vi "Dashboard.vi"() -> ()   [LabVIEW 2013]
uses:
  2014 Robot Project/Robot Global Data.vi
  <vilib>/sound2/lvsound2.llb/Sound File Read Open.vi
  <vilib>/sound2/lvsound2.llb/Sound File Read (DBL).vi
panel:
  out "Feeder":bool
  out "InvertDrive":bool
  out "ThumpFire":bool
  out "ThumpHigh":bool
  out "ThumpLow":bool
  out "DownLimit":bool
  out "DownLimit 2":bool
  out "Center":bool
  out "UpLimit 2":bool
  out "UpLimit":bool
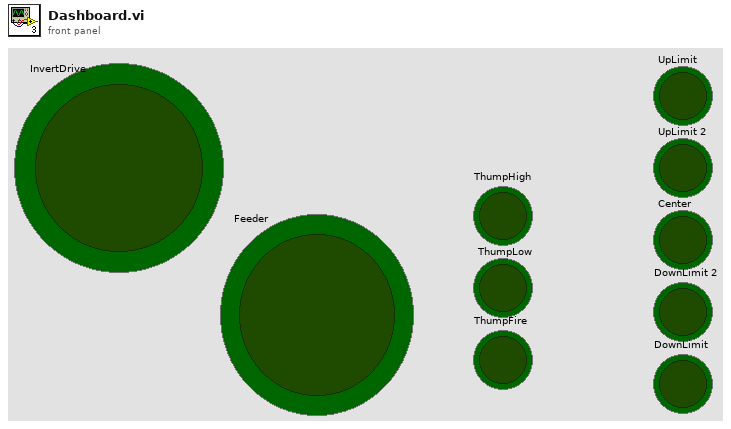
[diagram p1: front panel]
types:
  T1 = cluster{"UpLimit":bool, "Up2":bool, "Center":bool, "Down2":bool, "DownLimit":bool, "ThumpState":dbl, "ShifterState":bool, "FeederState":bool}
  T2 = cluster{"Competition mode":bool, "Robot Link":bool, "Autonomous":bool, "Enabled":bool, "E-Stop":bool, "Simulated":bool, "TestMode":bool, "Docked Window":bool}
  T3 = typedef "Sound File Refnum.ctl" = refnum<file>
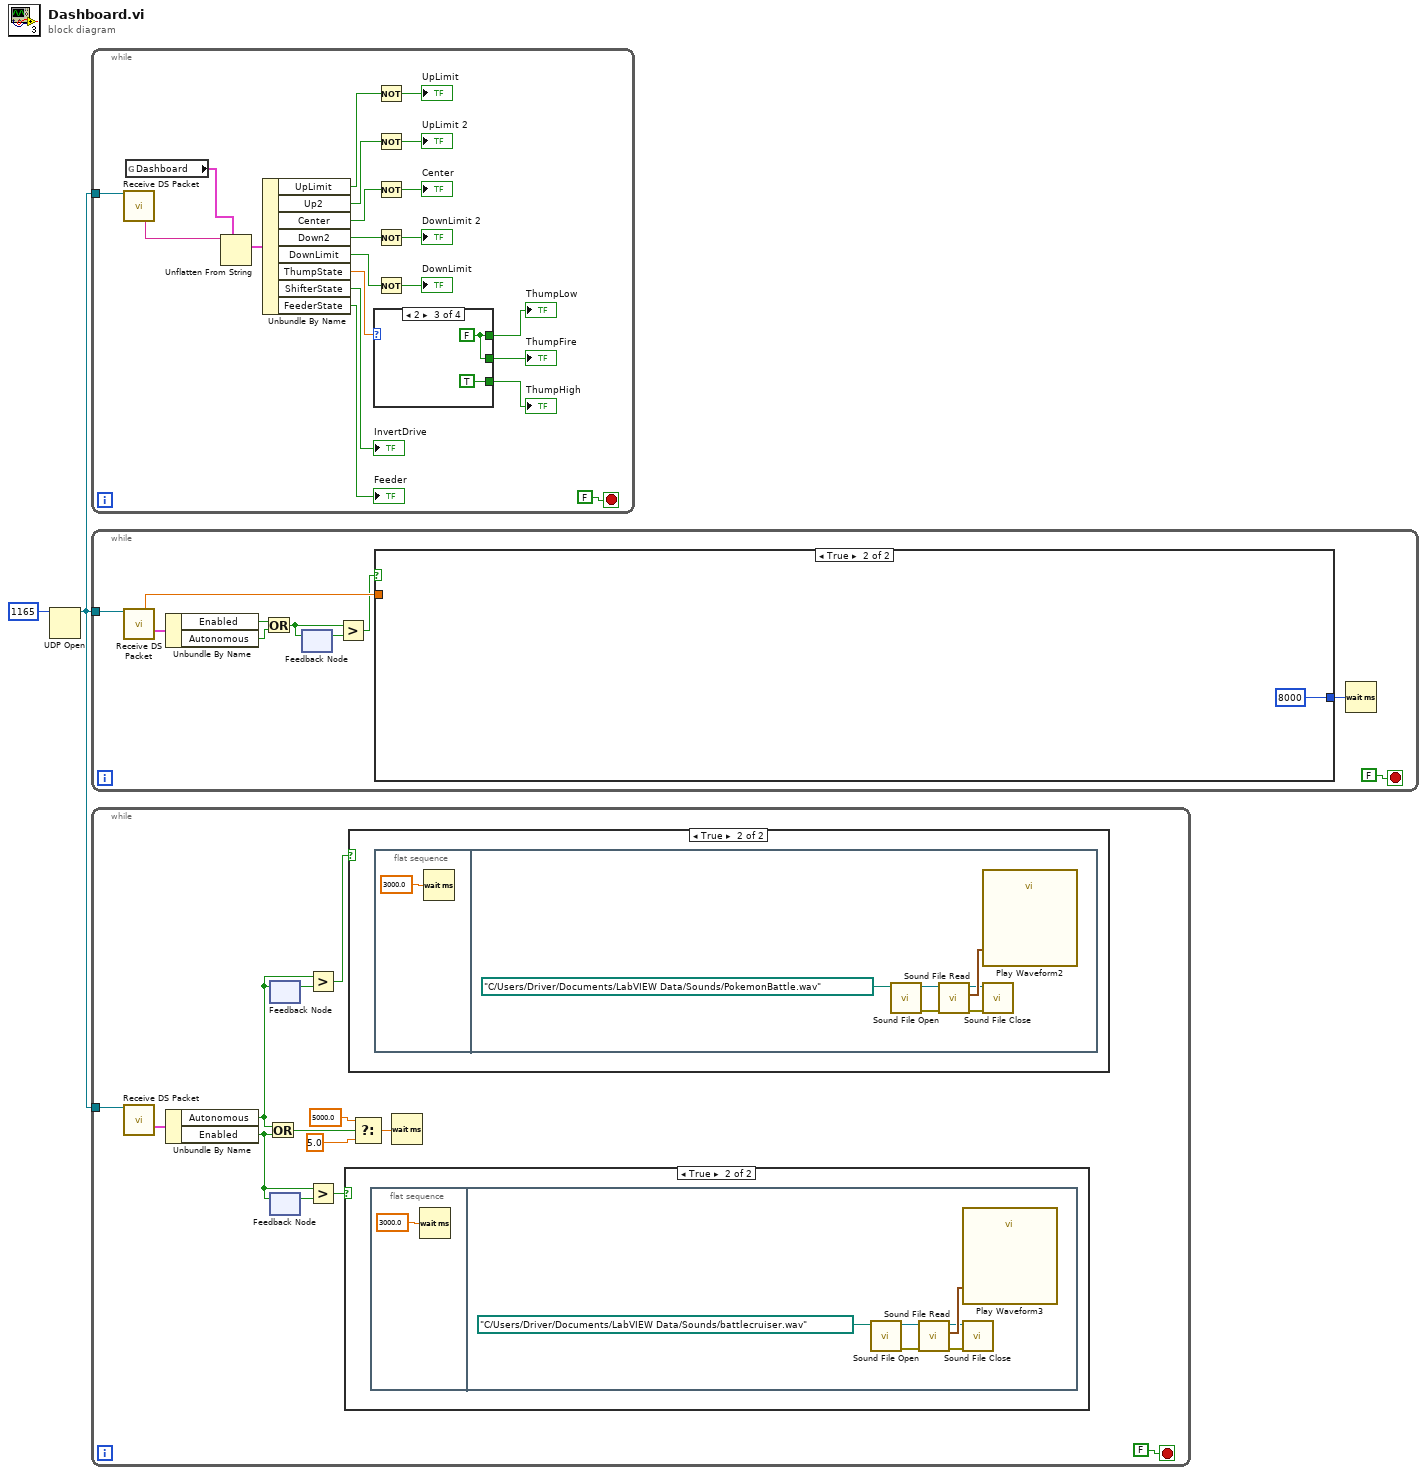
[diagram p0: block diagram]
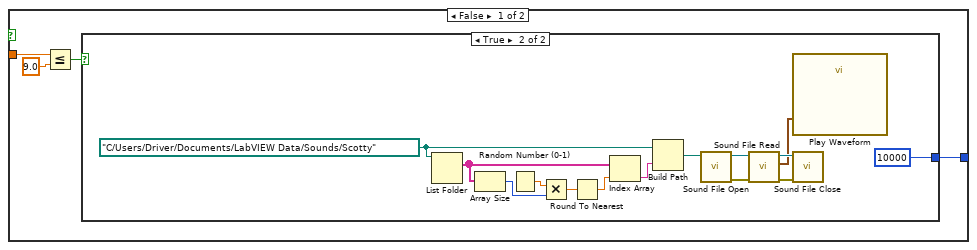
[diagram p4: hidden frame]
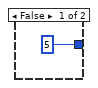
[diagram p5: hidden frame]
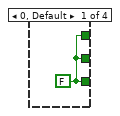
[diagram p6: hidden frame]
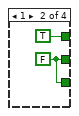
[diagram p7: hidden frame]
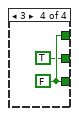
[diagram p8: hidden frame]
diagram:
  n1 = UDP Open(11:u16 1165 ("port")) -> (port=w1:refnum<k16>)  [unwired: 4 in, 2 out]
  n2 = while {
    tunnel: w1 -> [w23]
    stop <- FALSE stop-if-true
    n3 = call "Receive DS Packet.vi"("Recv Socket"=w23) -> ("High Priority User Data"=w22:string)  [unwired: 5 in, 9 out]
    n4 = global read "Robot Global Data.vi" "Dashboard"() -> (w20:T1)
    n5 = Unflatten From String(type=w20, binary string=w22) -> (value=w19:T1)  [unwired: 3 in, 2 out]
    n6 = Unbundle By Name(w19) -> ("UpLimit"=w7:bool, "Up2"=w6:bool, "Center"=w5:bool, "Down2"=w4:bool, "DownLimit"=w3:bool, "ThumpState"=w16:dbl, "ShifterState"=→"InvertDrive":bool, "FeederState"=→"Feeder":bool)
    n7 = case shown="2" w16 {
      tunnel: [w24 w26 TRUE w30] -> w15
      tunnel: [w24 TRUE w28 w30] -> w14
      tunnel: [w24 w26 w28 TRUE] -> w13
      frame 0, Default {
        w24 = FALSE
      }
      frame 1 {
        w26 = FALSE
      }
      frame 2 {
        w28 = FALSE
      }
      frame 3 {
        w30 = FALSE
      }
    }
    "ThumpHigh" <- w15
    "ThumpFire" <- w13
    "ThumpLow" <- w14
    n8 = Not(x=w7) -> (.not. x?=→"UpLimit":bool)
    n9 = Not(x=w6) -> (.not. x?=→"UpLimit 2":bool)
    n10 = Not(x=w5) -> (.not. x?=→"Center":bool)
    n11 = Not(x=w4) -> (.not. x?=→"DownLimit 2":bool)
    n12 = Not(x=w3) -> (.not. x?=→"DownLimit":bool)
  }
  n13 = while {
    tunnel: w1 -> [w40]
    stop <- FALSE stop-if-true
    n14 = call "Receive DS Packet.vi"("Recv Socket"=w40) -> ("Battery"=w39:sgl, "Status"=w36:T2)  [unwired: 5 in, 8 out]
    n15 = Unbundle By Name(w36) -> ("Enabled"=w33:bool, "Autonomous"=w32:bool)
    n16 = Or(x=w33, y=w32) -> (x .or. y?=w31:bool)
    n17 = feedback-in #1(w31) -> ()
    n18 = feedback #1() -> (w35:bool)  [unwired: 1 in]
    n19 = Greater?(x=w31, y=w35) -> (0:w34:bool)
    n20 = case shown="True" w34 {
      tunnel: w39 -> [w42 _]
      tunnel: [w41 8000] -> w38
      frame False {
        n21 = Less Or Equal?(x=w42, y=sgl 9.0) -> (x <= y?=w43:bool)
        n22 = case shown="True" w43 {
          tunnel: [5 10000] -> w41
          frame False {
          }
          frame True {
            w54 = path "C:/Users/Driver/Documents/LabVIEW Data/Sounds/Scotty" ("path")
            n23 = List Folder(path=w54) -> (filenames=w55:string[])  [unwired: 3 in, 3 out]
            n24 = Array Size(array=w55) -> (size(s)=w58:i32)
            n25 = Random Number (0-1)() -> (number: 0 to 1=w59:dbl)
            n26 = Multiply(x=w59, y=w58) -> (x*y=w57:dbl)
            n27 = Round To Nearest(number=w57) -> (nearest integer value=w56:dbl)
            n28 = Index Array(array=w55, index=w56) -> (element=w53:string)
            n29 = Build Path(base path=w54, name or relative path=w53) -> (appended path=w52:path)
            n30 = call-poly <vilib>:"Sound File Open.vi"("path"=w52) -> ("error out"=w48:errorcluster, "sound file refnum"=w51:T3)  [unwired: 9 in]
            n31 = call-poly <vilib>:"Sound File Read.vi"("error in (no error)"=w48, "sound file refnum"=w51) -> ("error out"=w49:errorcluster, "data"=w47:waveform(dbl)[], "sound file refnum out"=w50:T3)  [unwired: 5 in, 2 out]
            n32 = call "Play Waveform"("Data"=w47) -> ()  [unwired: 18 in, 1 out]
            n33 = call <vilib>:"Sound File Close.vi"("error in (no error)"=w49, "sound file refnum"=w50) -> ()  [unwired: 9 in, 1 out]
          }
        }
      }
      frame True {
      }
    }
    n34 = Wait (ms)(milliseconds to wait=w38) -> ()  [unwired: 1 out]
  }
  n35 = while {
    tunnel: w1 -> [w61]
    stop <- FALSE stop-if-true
    n36 = call "Receive DS Packet.vi"("Recv Socket"=w61) -> ("Status"=w73:T2)  [unwired: 5 in, 9 out]
    n37 = Unbundle By Name(w73) -> ("Autonomous"=w67:bool, "Enabled"=w66:bool)
    n38 = Or(x=w67, y=w66) -> (x .or. y?=w65:bool)
    n39 = feedback #2() -> (w72:bool)  [unwired: 1 in]
    n40 = feedback-in #2(w67) -> ()
    n41 = feedback #3() -> (w69:bool)  [unwired: 1 in]
    n42 = feedback-in #3(w66) -> ()
    n43 = Greater?(x=w67, y=w72) -> (0:w70:bool)
    n44 = Greater?(x=w66, y=w69) -> (0:w68:bool)
    n45 = case shown="True" w68 {
      frame False {
      }
      frame True {
        n46 = flat-sequence {
          frame #0 {
            n47 = Wait (ms)(milliseconds to wait=3000.0 ("t")) -> ()  [unwired: 1 out]
          }
          frame #1 {
            n48 = call-poly <vilib>:"Sound File Open.vi"("path"=path "C:/Users/Driver/Documents/LabVIEW Data/Sounds/battlecruiser.wav") -> ("error out"=w78:errorcluster, "sound file refnum"=w75:T3)  [unwired: 9 in]
            n49 = call-poly <vilib>:"Sound File Read.vi"("error in (no error)"=w78, "sound file refnum"=w75) -> ("error out"=w77:errorcluster, "data"=w79:waveform(dbl)[], "sound file refnum out"=w76:T3)  [unwired: 5 in, 2 out]
            n50 = call "Play Waveform3"("Data"=w79) -> ()  [unwired: 18 in, 1 out]
            n51 = call <vilib>:"Sound File Close.vi"("error in (no error)"=w77, "sound file refnum"=w76) -> ()  [unwired: 9 in, 1 out]
          }
        }
      }
    }
    n52 = case shown="True" w70 {
      frame False {
      }
      frame True {
        n53 = flat-sequence {
          frame #0 {
            n54 = Wait (ms)(milliseconds to wait=3000.0 ("t")) -> ()  [unwired: 1 out]
          }
          frame #1 {
            n55 = call-poly <vilib>:"Sound File Open.vi"("path"=path "C:/Users/Driver/Documents/LabVIEW Data/Sounds/PokemonBattle.wav") -> ("error out"=w85:errorcluster, "sound file refnum"=w82:T3)  [unwired: 9 in]
            n56 = call-poly <vilib>:"Sound File Read.vi"("error in (no error)"=w85, "sound file refnum"=w82) -> ("error out"=w84:errorcluster, "data"=w86:waveform(dbl)[], "sound file refnum out"=w83:T3)  [unwired: 5 in, 2 out]
            n57 = call "Play Waveform2"("Data"=w86) -> ()  [unwired: 18 in, 1 out]
            n58 = call <vilib>:"Sound File Close.vi"("error in (no error)"=w84, "sound file refnum"=w83) -> ()  [unwired: 9 in, 1 out]
          }
        }
      }
    }
    n59 = Select(t=5000.0, s=w65, f=5.0) -> (s? t:f=w64:dbl)
    n60 = Wait (ms)(milliseconds to wait=w64) -> ()  [unwired: 1 out]
  }
